vi "KH7008 COM Error Checker.vi"(2 "error in (no error)":errorcluster, 3 "String In":string) -> (0 "error out":errorcluster, 1 "String":string)   [LabVIEW 2019, in "Inst.Krohn-Hite-7008.lvclass"]
uses:
  Inst.Krohn-Hite-7008.lvclass
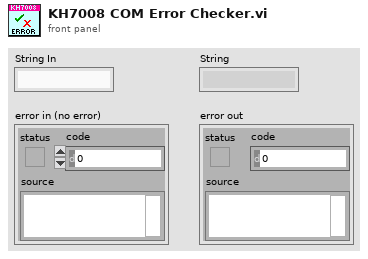
[diagram p1: front panel]
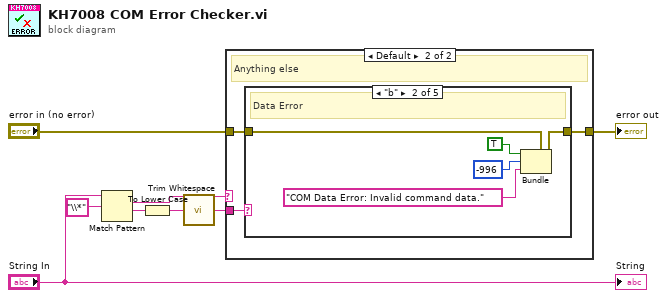
[diagram p0: block diagram]
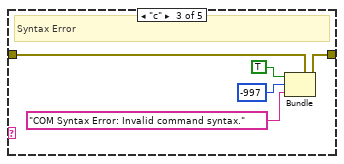
[diagram p4: hidden frame]
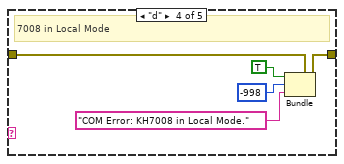
[diagram p5: hidden frame]
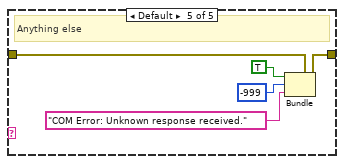
[diagram p6: hidden frame]
diagram:
  n1 = Match Pattern(string="String In", regular expression="\\*") -> (match substring=w2:string, after substring=w4:string)  [unwired: 1 in, 2 out]
  n2 = To Lower Case(string=w4) -> (all lower case string=w5:string)
  n3 = call <vilib>:"Trim Whitespace.vi"("string"=w5) -> ("trimmed string"=w6:string)  [unwired: 1 in]
  n4 = case shown="Default" w2 {
    tunnel: [w9 w12] -> w8
    tunnel: "error in (no error)" -> [w9 w11]
    tunnel: w6 -> [_ w10]
    frame "" {
    }
    frame Default {
      # "Anything else"
      n5 = case shown="\"b\"" w10 {
        tunnel: w11 -> [w13 w18 w23 w28 w30]
        tunnel: [w13 w14 w19 w24 w29] -> w12
        frame "a" {
          # "Data Ok, No errors"
        }
        frame "b" {
          # "Data Error"
          n6 = Bundle(cluster=w18, "status"=TRUE, "code"=-996, "source"="COM Data Error: Invalid command data.") -> (w14:errorcluster)
        }
        frame "c" {
          # "Syntax Error"
          n7 = Bundle(cluster=w23, "status"=TRUE, "code"=-997, "source"="COM Syntax Error: Invalid command syntax.") -> (w19:errorcluster)
        }
        frame "d" {
          # "7008 in Local Mode"
          n8 = Bundle(cluster=w28, "status"=TRUE, "code"=-998, "source"="COM Error: KH7008 in Local Mode.") -> (w24:errorcluster)
        }
        frame Default {
          # "Anything else"
          n9 = Bundle(cluster=w30, "status"=TRUE, "code"=-999, "source"="COM Error: Unknown response received.") -> (w29:errorcluster)
        }
      }
    }
  }
  "error out" <- w8
  "String" <- "String In"
